vi "KE6221 -- Execute PDelta Meas.vi"(0 "6221 Resource In":refnum<visa-resource-name>, 1 "Check For SCPI Errors? (T)":bool=TRUE, 5 "2812 -A Params In":T18={"Auto Range?"=FALSE, "Man / Selected\nRange"=enum."10mV", "Enable Digital\nFilter?"=FALSE, "Filter Type"=enum."Moving", "Filter Count"=10, "Filter\nWindow (%)"=0.01, "Enable Analog\nFilter?"=FALSE, "NPLCs"=5} {"Filter\nWindow (%)" min=0.0 max=10.0 step=0.01 format="%.2f"; "Filter Count" min=1 max=100; "NPLCs" min=1 max=10}, 7 "Pulsed Delta Mode Params In":T3={"High Level (A)"=0.001, "Low Level (A)"=0.0, "Pulse Width (s)"=0.00011, "Source Delay (s)"=6e-05, "Num Cycles Mode"=enum."Finite Count", "Finite Count"=10, "Ranging Mode"=enum."Best", "Num Low Meas Per Cycle"=enum."1", "Pulse Period (Num PLCs)"=5, "Pulse Sweep Mode Enabled?"=FALSE} {"Pulse Period (Num PLCs)" min=5 max=999990; "Source Delay (s)" min=1.6e-05 max=0.011966 format="%.3p"; "Pulse Width (s)" min=5e-05 max=0.012 format="%.3p"; "Finite Count" min=2 max=65536; "Low Level (A)" min=-0.105 max=0.0 format="%.3p"; "High Level (A)" min=0.0 max=0.105 format="%.3p"}, 9 "Meas Units":T2, 11 "error in (no error)":errorcluster, 12 "Power Meas Type":T1, 13 "Timeout (20000 ms)":u32=20000) -> (4 "6221 Resource Out (dupl)":refnum<visa-resource-name>, 6 "2812 -A Params Out":T18={"Auto Range?"=FALSE, "Man / Selected\nRange"=enum."10mV", "Enable Digital\nFilter?"=FALSE, "Filter Type"=enum."Moving", "Filter Count"=10, "Filter\nWindow (%)"=0.01, "Enable Analog\nFilter?"=FALSE, "NPLCs"=5} {"Filter\nWindow (%)" min=0.0 max=10.0 step=0.01 format="%.2f"; "Filter Count" min=1 max=100; "NPLCs" min=1 max=60}, 8 "Pulsed Delta Mode Params Out":T3={"High Level (A)"=0.001, "Low Level (A)"=0.0, "Pulse Width (s)"=0.00011, "Source Delay (s)"=1.6e-05, "Num Cycles Mode"=enum."Finite Count", "Finite Count"=1, "Ranging Mode"=enum."Best", "Num Low Meas Per Cycle"=enum."1", "Pulse Period (Num PLCs)"=5, "Pulse Sweep Mode Enabled?"=FALSE} {"Pulse Period (Num PLCs)" min=5 max=999990; "Source Delay (s)" min=1.6e-05 max=0.011966 format="%.3p"; "Pulse Width (s)" min=5e-05 max=0.012 format="%.3p"; "Finite Count" min=1 max=65536; "Low Level (A)" min=-0.105 max=0.0 format="%.3p"; "High Level (A)" min=0.0 max=0.105 format="%.3p"}, 10 "Timeout?":bool, 14 "Execution Time":dbl, 15 "error out":errorcluster)   [LabVIEW 2019, in "Keithley 622x.lvlib"]
doc: "Used to set up and execute a Pulsed Delta Mode measurement. This VI accepts setup parameters for both the 2182/2182A and the 6221 instruments. Note that the 6220 is incapable of supplying the current pulses, hence this VI should only be used with a 6221."
uses:
  Keithley 622x.lvlib
  Configure/2182 -A/Low Level/Typedefs/KE2182 -- Voltage Ranges.ctl
  Configure/2182 -A/Low Level/Typedefs/KE2182 -- Filter Type.ctl
  Configure/2182 -A/Low Level/Typedefs/KE2182 -- Filter Count.ctl
  Configure/2182 -A/Low Level/Typedefs/KE2182 -- Filter Window.ctl
  Configure/2182 -A/Low Level/Typedefs/KE2182 -- NPLCs.ctl
  Configure/Delta PDelta DCon Modes/Typedefs/KE6221 -- PDelta Mode Params.ctl
  Configure/Delta PDelta DCon Modes/Low Level/Typedefs/KE622x -- Delta PDelta Mode High Level.ctl
  Configure/Delta PDelta DCon Modes/Low Level/Typedefs/KE622x -- Delta PDelta Mode Low Level.ctl
  Configure/Delta PDelta DCon Modes/Low Level/Typedefs/KE6221 -- PDelta Mode Pulse Width.ctl
  Configure/Delta PDelta DCon Modes/Low Level/Typedefs/KE6221 -- PDelta Mode Source Delay.ctl
  Configure/Delta PDelta DCon Modes/Low Level/Typedefs/KE622x -- Delta PDelta Mode Num Cycles Mode.ctl
  Configure/Delta PDelta DCon Modes/Low Level/Typedefs/KE622x -- Delta PDelta Mode Num Cycles.ctl
  Configure/Delta PDelta DCon Modes/Low Level/Typedefs/KE6221 -- PDelta Mode Ranging Mode.ctl
  Configure/Delta PDelta DCon Modes/Low Level/Typedefs/KE6221 -- PDelta Mode Num Low Meas.ctl
  Configure/Delta PDelta DCon Modes/Low Level/Typedefs/KE6221 -- PDelta Mode Pulse Period.ctl
  Configure/Units/Typedefs/KE622x -- Voltage Meas Units.ctl
  Configure/Units/Typedefs/KE6221 -- PDelta Power Meas Type.ctl
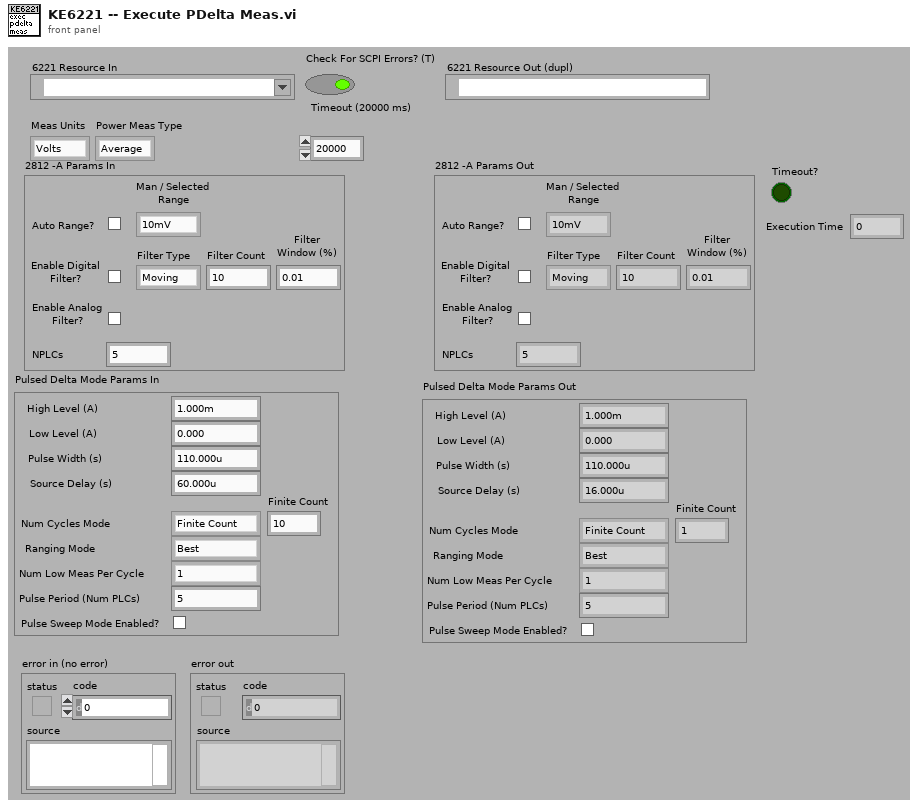
[diagram p1: front panel]
types:
  T1 = typedef "Keithley 622x.lvlib/KE6221 -- PDelta Power Meas Type.ctl" = enum16{"Average", "Peak"}
  T2 = typedef "Keithley 622x.lvlib/KE622x -- Voltage Meas Units.ctl" = enum16{"Volts", "Ohms", "Watts", "Siemens"}
  T3 = typedef "Keithley 622x.lvlib/KE6221 -- PDelta Mode Params.ctl" = cluster{"High Level (A)":T4, "Low Level (A)":T5, "Pulse Width (s)":T6, "Source Delay (s)":T7, "Num Cycles Mode":T8, "Finite Count":T9, "Ranging Mode":T10, "Num Low Meas Per Cycle":T11, "Pulse Period (Num PLCs)":T12, "Pulse Sweep Mode Enabled?":bool}
  T4 = typedef "Keithley 622x.lvlib/KE622x -- Delta PDelta Mode High Level.ctl" = dbl
  T5 = typedef "Keithley 622x.lvlib/KE622x -- Delta PDelta Mode Low Level.ctl" = dbl
  T6 = typedef "Keithley 622x.lvlib/KE6221 -- PDelta Mode Pulse Width.ctl" = dbl
  T7 = typedef "Keithley 622x.lvlib/KE6221 -- PDelta Mode Source Delay.ctl" = dbl
  T8 = typedef "Keithley 622x.lvlib/KE622x -- Delta PDelta Mode Num Cycles Mode.ctl" = enum16{"Finite Count", "Infinite"}
  T9 = typedef "Keithley 622x.lvlib/KE622x -- Delta PDelta Mode Num Cycles.ctl" = u32
  T10 = typedef "Keithley 622x.lvlib/KE6221 -- PDelta Mode Ranging Mode.ctl" = enum16{"Best", "Fixed"}
  T11 = typedef "Keithley 622x.lvlib/KE6221 -- PDelta Mode Num Low Meas.ctl" = enum16{"1", "2"}
  T12 = typedef "Keithley 622x.lvlib/KE6221 -- PDelta Mode Pulse Period.ctl" = u32
  T13 = typedef "Keithley 622x.lvlib/KE2182 -- Voltage Ranges.ctl" = enum16{"10mV", "100mV", "1V", "10V", "100V"}
  T14 = typedef "Keithley 622x.lvlib/KE2182 -- Filter Type.ctl" = enum16{"Moving", "Repeat"}
  T15 = typedef "Keithley 622x.lvlib/KE2182 -- Filter Count.ctl" = u32
  T16 = typedef "Keithley 622x.lvlib/KE2182 -- Filter Window.ctl" = dbl
  T17 = typedef "Keithley 622x.lvlib/KE2182 -- NPLCs.ctl" = u32
  T18 = cluster{"Auto Range?":bool, "Man / Selected\nRange":T13, "Enable Digital\nFilter?":bool, "Filter Type":T14, "Filter Count":T15, "Filter\nWindow (%)":T16, "Enable Analog\nFilter?":bool, "NPLCs":T17}
  T19 = typedef "Keithley 622x.lvlib/KE622x -- Meas Event Reg State.ctl" = cluster{"B0, ROF:  KE2182A Delta Reading Overflow Event?":bool, "B1, Int:  Interlock OK Event?":bool, "B2, Temp:  Over Temperature Event?":bool, "B3, Comp:  Compliance Event?":bool, "B5, RAV:  Delta Reading Available Event?":bool, "B6, TN:  User Defined Reading Number Stored In Buffer Event?":bool, "B7, BAV:  At Least 2 Readings Stored In Buffer Event?":bool, "B12, BQF:  Buffer Quarter Full Event?":bool, "B8, BHF:  Buffer Half Full Event?":bool, "B13, B3QF:  Buffer 3/4 Full Event?":bool, "B9, BFL:  Buffer Full Event?":bool}
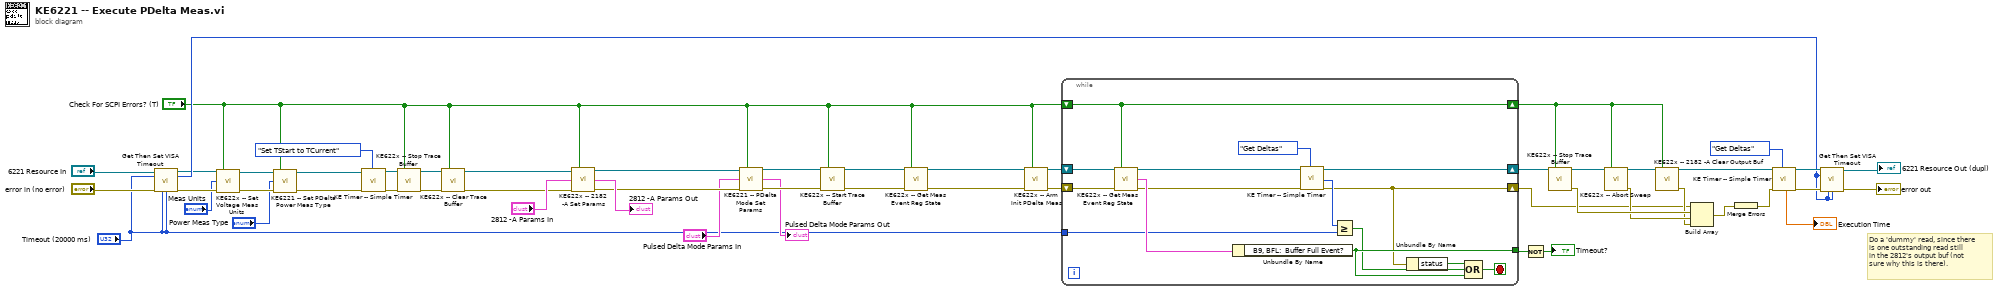
[diagram p0: block diagram]
diagram:
  # "Do a 'dummy' read, since there\nis one outstanding read still\nin the 2812's output buf (not\nsure why this is there)."
  n1 = call "Get Then Set VISA Timeout.vi"("VISA Resource Name In"="6221 Resource In", "New Timeout (msecs)"="Timeout (20000 ms)", "error in (no error)"="error in (no error)", "Max Timeout (300 secs)"="Timeout (20000 ms)", "Min Timeout (3 secs)"="Timeout (20000 ms)") -> ("VISA Resource Name Out (dupl)"=w9:refnum<visa-resource-name>, "Old Timeout (msecs)"=w10:u32, "error out"=w8:errorcluster)  [unwired: 7 in, 1 out]
  n2 = call "KE622x -- Set Voltage Meas Units.vi"("Resource In"=w9, "Check For SCPI Errors? (T)"="Check For SCPI Errors? (T)", "Voltage Meas Units"="Meas Units", "error in (no error)"=w8) -> ("Resource Out (dupl)"=w6:refnum<visa-resource-name>, "error out"=w5:errorcluster)  [unwired: 10 in]
  n3 = call "KE6221 -- Set PDelta Power Meas Type.vi"("6221 Resource In"=w6, "Check For SCPI Errors? (T)"="Check For SCPI Errors? (T)", "Power Meas Type"="Power Meas Type", "error in (no error)"=w5) -> ("6221 Resource Out (dupl)"=w2:refnum<visa-resource-name>, "error out"=w1:errorcluster)  [unwired: 10 in]
  n4 = call "KE Timer -- Simple Timer.vi"("Resource In"=w2, "error in (no error)"=w1, "Action"=enum16{"Set TStart to TCurrent", "Get Deltas"}."Set TStart to TCurrent") -> ("Resource Out (dupl)"=w31:refnum<visa-resource-name>, "error out (dupl)"=w30:errorcluster)  [unwired: 7 in, 8 out]
  n5 = call "KE622x -- Stop Trace Buffer.vi"("Resource In"=w31, "Check For SCPI Errors? (T)"="Check For SCPI Errors? (T)", "error in (no error)"=w30) -> ("Resource Out (dupl)"=w49:refnum<visa-resource-name>, "error out"=w48:errorcluster)  [unwired: 11 in]
  n6 = call "KE622x -- Clear Trace Buffer.vi"("Resource In"=w49, "Check For SCPI Errors? (T)"="Check For SCPI Errors? (T)", "error in (no error)"=w48) -> ("Resource Out (dupl)"=w27:refnum<visa-resource-name>, "error out"=w26:errorcluster)  [unwired: 11 in]
  n7 = call "KE622x -- 2182 -A Set Params.vi"("622x Resource In"=w27, "Check For SCPI Errors? (T)"="Check For SCPI Errors? (T)", "2812 -A Params In"="2812 -A Params In", "error in (no error)"=w26) -> ("622x Resource Out (dupl)"=w51:refnum<visa-resource-name>, "2812 -A Params Out"=→"2812 -A Params Out":T18, "error out"=w50:errorcluster)  [unwired: 9 in]
  n8 = call "KE6221 -- PDelta Mode Set Params.vi"("6221 Resource In"=w51, "Check For SCPI Errors? (T)"="Check For SCPI Errors? (T)", "Pulsed Delta Mode Params In"="Pulsed Delta Mode Params In", "error in (no error)"=w50) -> ("6221 Resource Out (dupl)"=w47:refnum<visa-resource-name>, "Pulsed Delta Mode Params Out"=→"Pulsed Delta Mode Params Out":T3, "error out"=w46:errorcluster)  [unwired: 9 in]
  n9 = call "KE622x -- Start Trace Buffer.vi"("Resource In"=w47, "Check For SCPI Errors? (T)"="Check For SCPI Errors? (T)", "error in (no error)"=w46) -> ("Resource Out (dupl)"=w44:refnum<visa-resource-name>, "error out"=w45:errorcluster)  [unwired: 11 in]
  n10 = call "KE622x -- Get Meas Event Reg State.vi"("VISA Resource In"=w44, "Error Query (T)?"="Check For SCPI Errors? (T)", "error in (no error)"=w45) -> ("VISA Resource Out (dupl)"=w29:refnum<visa-resource-name>, "error out"=w28:errorcluster)  [unwired: 10 in, 1 out]
  n11 = call "KE622x -- Arm Init PDelta Meas.vi"("Resource In"=w29, "Check For SCPI Errors? (T)"="Check For SCPI Errors? (T)", "error in (no error)"=w28) -> ("Resource Out (dupl)"=w41:refnum<visa-resource-name>, "error out"=w42:errorcluster)  [unwired: 11 in]
  n12 = while {
    shift-right: [w56] -> w18
    shift-left: w42 -> [w68]
    shift-right: [w58] -> w38
    shift-left: w41 -> [w67]
    tunnel: [w60] -> w40
    shift-right: [w57] -> w35
    shift-left: "Check For SCPI Errors? (T)" -> [w57]
    tunnel: "Timeout (20000 ms)" -> [w54]
    stop <- w61 stop-if-true
    n13 = call "KE622x -- Get Meas Event Reg State.vi"("VISA Resource In"=w67, "Error Query (T)?"=w57, "error in (no error)"=w68) -> ("VISA Resource Out (dupl)"=w64:refnum<visa-resource-name>, "KE622x Meas Event Reg"=w66:T19, "error out"=w65:errorcluster)  [unwired: 10 in]
    n14 = Unbundle By Name(w66) -> ("B9, BFL:  Buffer Full Event?"=w60:bool)
    n15 = call "KE Timer -- Simple Timer.vi"("Resource In"=w64, "error in (no error)"=w65, "Action"=enum16{"Set TStart to TCurrent", "Get Deltas"}."Get Deltas") -> ("Resource Out (dupl)"=w58:refnum<visa-resource-name>, "TCurrent - TStart (ms)"=w62:u32, "error out (dupl)"=w56:errorcluster)  [unwired: 7 in, 7 out]
    n16 = Greater Or Equal?(x=w62, y=w54) -> (x >= y?=w59:bool)
    n17 = Unbundle By Name(w56) -> ("status"=w55:bool)
    n18 = Compound Arithmetic op=OR(w55, w59, w60) -> (w61:bool)
  }
  n19 = Not(x=w40) -> (.not. x?=→"Timeout?":bool)
  n20 = call "KE622x -- Stop Trace Buffer.vi"("Resource In"=w38, "Check For SCPI Errors? (T)"=w35) -> ("Resource Out (dupl)"=w37:refnum<visa-resource-name>, "error out"=w23:errorcluster)  [unwired: 12 in]
  n21 = call "KE622x -- Abort Sweep.vi"("Resource In"=w37, "Check For SCPI Errors? (T)"=w35) -> ("Resource Out (dupl)"=w36:refnum<visa-resource-name>, "error out"=w22:errorcluster)  [unwired: 12 in]
  n22 = call "KE622x -- 2182 -A Clear Output Buf.vi"("622x Resource In"=w36, "Check For SCPI Errors? (T)"=w35) -> ("622x Resource Out (dupl)"=w34:refnum<visa-resource-name>, "error out"=w21:errorcluster)  [unwired: 11 in, 1 out]
  n23 = Build Array(w18, w23, w22, w21) -> (w20:errorcluster[])
  n24 = Merge Errors(w20) -> (w19:errorcluster)
  n25 = call "KE Timer -- Simple Timer.vi"("Resource In"=w34, "error in (no error)"=w19, "Action"=enum16{"Set TStart to TCurrent", "Get Deltas"}."Get Deltas") -> ("TCurrent - TStart (s)"=→"Execution Time":dbl, "Resource Out (dupl)"=w17:refnum<visa-resource-name>, "error out (dupl)"=w16:errorcluster)  [unwired: 7 in, 7 out]
  n26 = call "Get Then Set VISA Timeout.vi"("VISA Resource Name In"=w17, "New Timeout (msecs)"=w10, "error in (no error)"=w16, "Max Timeout (300 secs)"=w10, "Min Timeout (3 secs)"=w10) -> ("VISA Resource Name Out (dupl)"=→"6221 Resource Out (dupl)":refnum<visa-resource-name>, "error out"=→"error out":errorcluster)  [unwired: 7 in, 2 out]
